vi "RGBA to Color.vi"(1 "A":u8, 2 "B":u8, 3 "G":u8, 4 "R":u8) -> (0 "Color":u32(colorbox))   [LabVIEW 2023, in "Font Glyph Drawer Interface.lvlib"]
uses:
  Font Glyph Drawer Interface.lvlib
panel:
  out "result":u32 format="%.0x"
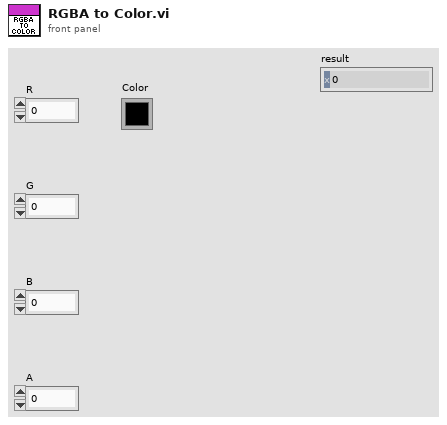
[diagram p1: front panel]
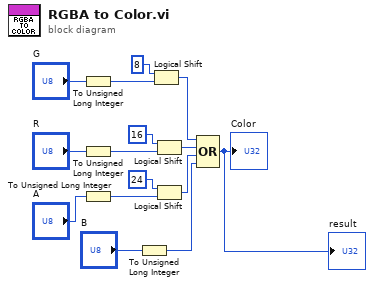
[diagram p0: block diagram]
diagram:
  n1 = To Unsigned Long Integer(number="G") -> (unsigned 32bit integer=w11:u32)
  n2 = To Unsigned Long Integer(number="R") -> (unsigned 32bit integer=w8:u32)
  n3 = To Unsigned Long Integer(number="A") -> (unsigned 32bit integer=w5:u32)
  n4 = To Unsigned Long Integer(number="B") -> (unsigned 32bit integer=w2:u32)
  n5 = Logical Shift(y=i16 8, x=w11) -> (x << y=w9:u32)
  n6 = Logical Shift(y=i16 16, x=w8) -> (x << y=w4:u32)
  n7 = Logical Shift(y=i16 24, x=w5) -> (x << y=w3:u32)
  n8 = Compound Arithmetic op=OR(w9, w4, w3, w2) -> (→"Color" →"result":u32)
